vi "UMLEditor ShowAggregationDialog.vi"(1 "graph":refnum<class "Graph.lvclass">, 2 "ClassAggregation":refnum<class "AbstractEdge.lvclass">, 5 "error in (no error)":errorcluster) -> (12 "Base class.bounds":T2 {"height" format="%.2f"; "width" format="%.2f"; "y" format="%.2f"; "x" format="%.2f"}, 15 "Show":bool, 16 "Remove":bool, 17 "StartEndNodes":T1, 19 "error out":errorcluster)   [LabVIEW 2014]
doc: "Gets current diagram values"
uses:
  <resource>/Framework/Providers/Open_GDS/UML/Graph_class/Graph.lvclass
  <resource>/Framework/Providers/Open_GDS/UML/AbstractEdge_class/AbstractEdge.lvclass
  <resource>/Framework/Providers/Open_GDS/UML/General/Rectangle/Rectangle Rectangle2D.ctl
  <resource>/Framework/Providers/Open_GDS/UML/AbstractNode_class/AbstractNode.lvclass
  <resource>/Framework/Providers/Open_GDS/UML/ClassNode_class/ClassNode.lvclass
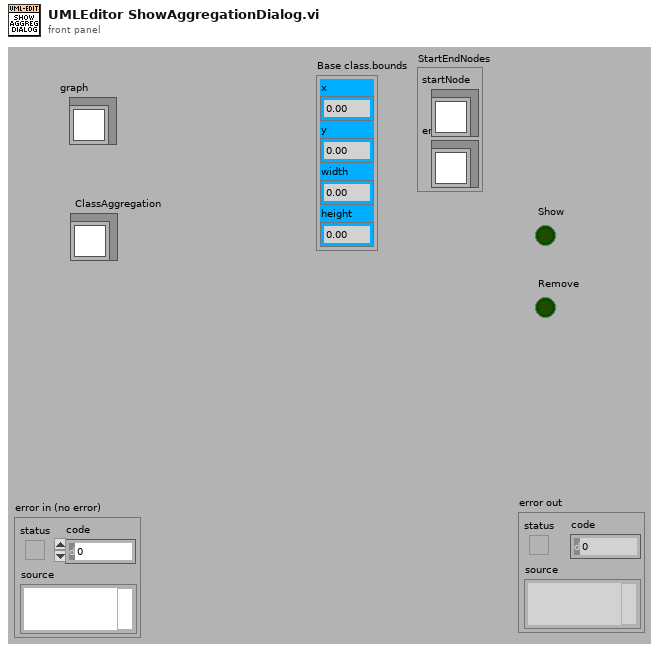
[diagram p1: front panel]
types:
  T1 = cluster{"startNode":refnum<class "AbstractNode.lvclass">, "endNode":refnum<class "AbstractNode.lvclass">}
  T2 = typedef "Rectangle Rectangle2D.ctl" = cluster{"x":dbl, "y":dbl, "width":dbl, "height":dbl}
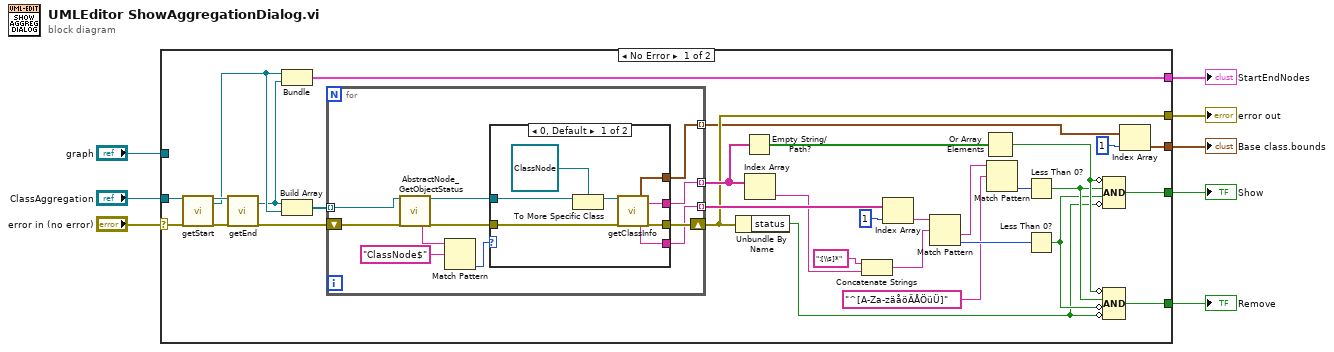
[diagram p0: block diagram]
diagram:
  n1 = case shown="No Error" "error in (no error)" {
    selector: "error in (no error)" -> [w39 w60]
    tunnel: [w16 w60] -> w4
    tunnel: "ClassAggregation" -> [w38 _]
    tunnel: "graph" -> [_ _]
    tunnel: [w37 _] -> w5
    tunnel: [w17 _] -> w3
    tunnel: [w13 _] -> w2
    tunnel: [w9 _] -> w1
    frame No Error {
      n2 = call-dynamic "getStart.vi"("reference"=w38, "error in (no error)"=w39) -> ("reference out"=w35:refnum<class "AbstractEdge.lvclass">, "startNode"=w11:refnum<class "AbstractNode.lvclass">, "error out"=w36:errorcluster)  [unwired: 14 in, 1 out]
      n3 = call-dynamic "getEnd.vi"("reference"=w35, "error in (no error)"=w36) -> ("endNode"=w10:refnum<class "AbstractNode.lvclass">, "error out"=w34:errorcluster)  [unwired: 14 in, 2 out]
      n4 = Bundle("startNode"=w11, "endNode"=w10) -> (w9:T1)  [unwired: 1 out]
      n5 = Build Array(w10, w11) -> (w33:refnum<class "AbstractNode.lvclass">[])
      n6 = for {
        tunnel: w33 -> [w43] mode=indexing
        shift-right: [w50] -> w16
        shift-left: w34 -> [w44]
        tunnel: [w42] -> w31 mode=indexing
        tunnel: [w41] -> w30 mode=indexing
        tunnel: [w40] -> w14 mode=indexing
        n7 = call <resource>:"AbstractNode_GetObjectStatus.vi"("reference in"=w43, "error in (no error)"=w44) -> ("Class name"=w48:string, "reference out"=w45:refnum<class "AbstractNode.lvclass">, "error out"=w46:errorcluster)  [unwired: 15 out]
        n8 = Match Pattern(string=w48, regular expression="ClassNode$") -> (offset past match=w47:i32)  [unwired: 4 out]
        n9 = case shown="0, Default" w47 {
          tunnel: w46 -> [w54 w59]
          tunnel: w45 -> [w53 _]
          tunnel: [w58 w59] -> w50
          tunnel: [w56 _] -> w41
          tunnel: [w57 _] -> w42
          tunnel: [w55 _] -> w40
          frame 0, Default {
            n10 = To More Specific Class(target class=refnum<class "ClassNode.lvclass"> refnum ("reference"), reference=w53) -> (specific class reference=w52:refnum<class "ClassNode.lvclass">)  [unwired: 1 in, 1 out]
            n11 = call-dynamic "getClassInfo.vi"("reference"=w52, "error in (no error)"=w54) -> ("Base class.bounds"=w55:T2, "attributes(string)"=w57:string, "className"=w56:string, "error out"=w58:errorcluster)  [unwired: 8 in, 6 out]
          }
          frame -1 {
          }
        }
      }
      n12 = Unbundle By Name(w16) -> ("status"=w15:bool)
      n13 = Empty String/Path?(string/path=w30) -> (empty?=w32:bool[])
      n14 = Index Array(array=w30) -> (element=w26:string)  [unwired: 1 in]
      n15 = Concatenate Strings(":[\\s]*" ("regular expression"), w26) -> (w25:string)
      n16 = Index Array(array=w31, index=1) -> (element=w28:string)
      n17 = Match Pattern(string=w28, regular expression=w25) -> (after substring=w23:string, offset past match=w24:i32)  [unwired: 3 out]
      n18 = Or Array Elements(Boolean array=w32) -> (logical OR=w20:bool)
      n19 = Match Pattern(string=w23, regular expression="^[A-Za-zäåöÄÅÖüÜ]") -> (offset past match=w21:i32)  [unwired: 4 out]
      n20 = Less Than 0?(x=w21) -> (x < 0?=w19:bool)
      n21 = Less Than 0?(x=w24) -> (x < 0?=w18:bool)
      n22 = Compound Arithmetic op=AND(invert w20, w19, w18, invert w15) -> (w37:bool)
      n23 = Compound Arithmetic op=AND(invert w20, w19, invert w18, invert w15) -> (w17:bool)
      n24 = Index Array(array=w14, index=1) -> (element=w13:T2)
    }
    frame Error {
    }
  }
  "error out" <- w4
  "Show" <- w5
  "Remove" <- w3
  "Base class.bounds" <- w2
  "StartEndNodes" <- w1
